vi "Update Rooms List.vi"(0 "Guest Manager UI in":refnum<class "Guest Manager UI.lvclass">, 5 "All Rooms":string[](array[string]), 7 "Available Rooms":string[](array[string]), 11 "error in (no error)":errorcluster) -> (4 "Guest Manager UI out":refnum<class "Guest Manager UI.lvclass">, 15 "error out":errorcluster)   [LabVIEW 2023, in "Guest Manager UI.lvlib" / "Guest Manager UI.lvclass"]
uses:
  Guest Manager UI.lvclass
  Guest Manager UI.lvclass/Guest Manager UI.ctl
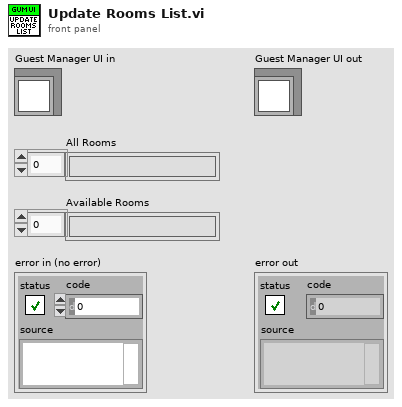
[diagram p1: front panel]
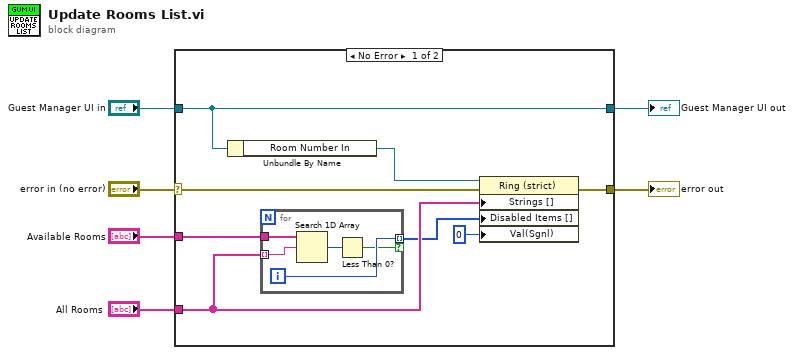
[diagram p0: block diagram]
diagram:
  n1 = case shown="No Error" "error in (no error)" {
    selector: "error in (no error)" -> [w14 w21]
    tunnel: [w13 w21] -> w5
    tunnel: [w12 w20] -> w3
    tunnel: "Guest Manager UI in" -> [w12 w20]
    tunnel: "All Rooms" -> [w9 _]
    tunnel: "Available Rooms" -> [w10 _]
    frame No Error {
      n2 = Unbundle By Name(w12) -> ("Room Number In"=w11:refnum<vi>)
      n3 = for {
        tunnel: w10 -> [w19]
        tunnel: w9 -> [w18] mode=indexing
        tunnel: [w16] -> w8 mode=indexing if=w15
        i -> [w16]
        n4 = Search 1D Array(1D array=w19, element=w18) -> (index of element=w17:i32)  [unwired: 1 in]
        n5 = Less Than 0?(x=w17) -> (x < 0?=w15:bool)
      }
      n6 = property class="Ring (strict)"(reference=w11, error in=w14, "Strings []"=w9, "Disabled Items []"=w8, "Val(Sgnl)"=u16 0 ("Value (Signaling)")) -> (error out=w13:errorcluster)  [unwired: 1 out]
    }
    frame Error {
    }
  }
  "error out" <- w5
  "Guest Manager UI out" <- w3
